vi "add_complete_overlay_pattern.vi"(5 "center radius":dbl, 6 "Color":u32(colorbox)=16448250, 7 "number of rings":i32, 9 "Image Name":string="alignment_overlay", 10 "Image Src":T1) -> (2 "Image Out":T1)   [LabVIEW 2011]
doc: "Creates Overlay pattern to help with the alignment of the setup. The input image is copied and a new memory space is create to hold the overlay image in order to keep the originally created pattern."
uses:
  <vilib>/vision/Image Controls.llb/IMAQ Image.ctl
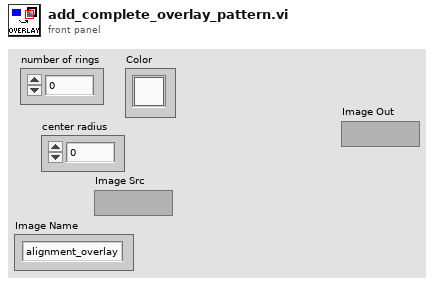
[diagram p1: front panel]
types:
  T1 = typedef "IMAQ Image.ctl" = refnum<image>
  T2 = cluster{"Desired Font (Application)":enum16{"User-specified Font", "Application Font", "System Font", "Dialog Font"}, "[User-specified Font]":cluster{"Font Name":string, "Size":i16, "Strikeout?":bool, "Italic?":bool, "Underline?":bool, "Outline?":bool, "Shadow?":bool, "Bold?":bool, "Rotation Angle":dbl}, "Horizontal Alignment":i16, "Vertical Alignment":i16}
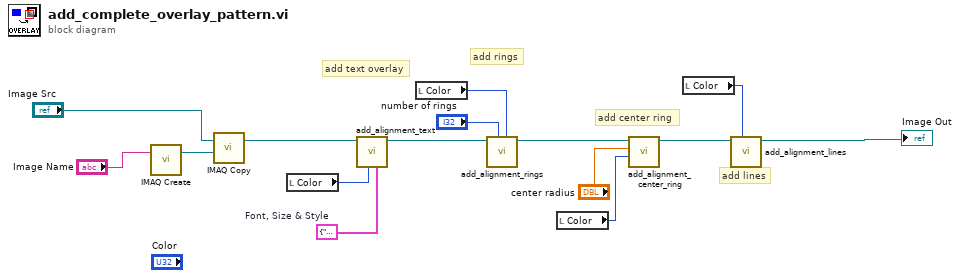
[diagram p0: block diagram]
diagram:
  w10 = T2 {"Desired Font (Application)"=enum."User-specified Font", "[User-specified Font]"={"Font Name"="Arial", "Size"=30, "Strikeout?"=FALSE, "Italic?"=FALSE, "Underline?"=FALSE, "Outline?"=FALSE, "Shadow?"=FALSE, "Bold?"=TRUE, "Rotation Angle"=0.0}, "Horizontal Alignment"=1, "Vertical Alignment"=2}  # Font, Size & Style
  # "add center ring"
  # "add lines"
  # "add rings"
  # "add text overlay"
  n1 = call "IMAQ Create"("Image Name"="Image Name") -> ("New Image"=w14:T1)  [unwired: 4 in, 1 out]
  n2 = call "IMAQ Copy"("Image Dst"=w14, "Image Src"="Image Src") -> ("Image Dst Out"=w15:T1)  [unwired: 4 in, 1 out]
  n3 = local read "Color"() -> (w9:u32)
  n4 = call "add_alignment_text.vi"("Font, Size & Style"=w10, "Color"=w9, "image in"=w15) -> ("image out"=w13:T1)  [unwired: 8 in]
  n5 = local read "Color"() -> (w4:u32)
  n6 = call "add_alignment_rings.vi"("Color"=w4, "number of rings"="number of rings", "Image in"=w13) -> ("Image Out"=w7:T1)  [unwired: 6 in]
  n7 = local read "Color"() -> (w6:u32)
  n8 = call "add_alignment_center_ring.vi"("Color"=w6, "center radius"="center radius", "Refnum in"=w7) -> ("Refnum out"=w11:T1)  [unwired: 8 in]
  n9 = local read "Color"() -> (w5:u32)
  n10 = call "add_alignment_lines.vi"("Color"=w5, "Image in"=w11) -> ("Image out"=→"Image Out":T1)  [unwired: 9 in]
